vi "Write Slow FPGA Telem to FIFO.vi"   [LabVIEW 2015]
uses:
  FPGA Telem for Slow Logging.ctl
  <vilib>/FPGAPlugInAG/Dynamic/niLvFpga_Close_Dynamic.vi
  <vilib>/rvi/errors/niLvFpgaAdjustHostInterfaceError.vi
  <vilib>/Utility/error.llb/Error Cluster From Error Code.vi
  Global Data.vi
  <vilib>/rvi/interface/common/dynamic/niFpgaDynamicAddResources.vi
  <vilib>/FPGAPlugInAG/sbRIO-9627/niLvFpga_Open_sbRIO-9627.vi
  <vilib>/rvi/interface/nirviCloseFPGA/nirviCloseFPGA.xnode
  <vilib>/rvi/interface/nirviReadWriteControl/nirviReadWriteControl.xnode
  <vilib>/rvi/interface/nirviOpenFPGA/nirviOpenFPGA.xnode
  FPGA Bitfiles/Latest.lvbitx
  <vilib>/NI_Real-Time Target Support.lvlib
  NiFpgaLv.dll
  <vilib>/rvi/interface/Simulation/niFpgaSimulationCallBeginRW.vi
types:
  T1 = cluster{"read mode":enum16{"polling", "blocking"}, "write mode":enum16{"polling", "blocking"}}
  T2 = typedef "FPGA Telem for Slow Logging.ctl" = cluster{"TSBRIO":fxp<+/-,16,9>, "VsbRIOSpply":fxp<+/-,25,6>, "bFPGALED":bool, "CPU Load":cluster{"Total (%)":dbl, "Time Critical (%)":dbl, "Timed Structures (%)":dbl, "High (%)":dbl, "Above Normal (%)":dbl, "Normal (%)":dbl, "Background (%)":dbl, "Idle (%)":dbl, "ISR (%)":dbl}, "Time Stamp":timestamp, "NLatiPhone":dbl, "NLongiPhone":dbl, "nGPSiPhone":dbl, "IHighCurrent":fxp<+/-,24,15>, "ILowCurrent":fxp<+/-,24,15>, "V5VSupply":fxp<+/-,24,5>, "tCurrentLap":u32, "tLastLap":u32, "NLap":u8, "bCoolantPumpEnable":bool, "bRTDSEnable":bool, "bTSMSInStatus":bool, "bPosAIREnable":bool, "bBMSOK":bool, "bIMDOK":bool, "bBSPDOK":bool, "bSBRIOOK2":bool, "bSBRIOOK1":bool, "bTSMSOutStatus":bool, "bMotorControllerEnable":bool, "Tire Diameter(m)":fxp<+,16,1>}
  T3 = typedef "NI_Real-Time Target Support.lvlib/RT CPU Load.ctl" = cluster{"Total (%)":dbl, "Time Critical (%)":dbl, "Timed Structures (%)":dbl, "High (%)":dbl, "Above Normal (%)":dbl, "Normal (%)":dbl, "Background (%)":dbl, "Idle (%)":dbl, "ISR (%)":dbl}
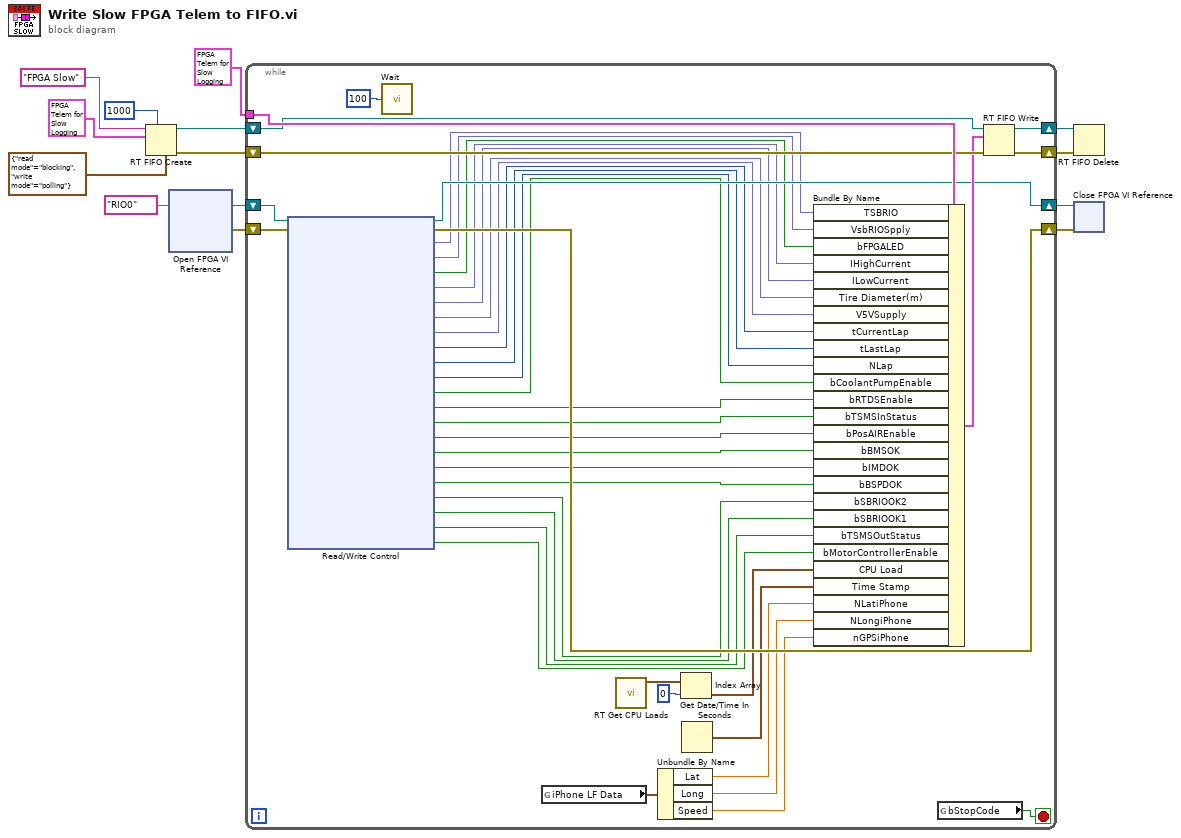
[diagram p0: block diagram]
diagram:
  n1 = RT FIFO Create(0:"FPGA Slow" ("name (unnamed)"), 1:T2 {"TSBRIO"=0.0, "VsbRIOSpply"=0.0, "bFPGALED"=FALSE, "CPU Load"={"Total (%)"=0.0, "Time Critical (%)"=0.0, "Timed Structures (%)"=0.0, "High (%)"=0.0, "Above Normal (%)"=0.0, "Normal (%)"=0.0, "Background (%)"=0.0, "Idle (%)"=0.0, "ISR (%)"=0.0}, "Time Stamp"=timestamp(0 s since 1904-01-01), "NLatiPhone"=0.0, "NLongiPhone"=0.0, "nGPSiPhone"=0.0, "IHighCurrent"=0.0, "ILowCurrent"=0.0, "V5VSupply"=-16.0, "tCurrentLap"=4, "tLastLap"=0, "NLap"=0, "bCoolantPumpEnable"=FALSE, "bRTDSEnable"=FALSE, "bTSMSInStatus"=FALSE, "bPosAIREnable"=FALSE, "bBMSOK"=TRUE, "bIMDOK"=TRUE, "bBSPDOK"=FALSE, "bSBRIOOK2"=FALSE, "bSBRIOOK1"=FALSE, "bTSMSOutStatus"=FALSE, "bMotorControllerEnable"=FALSE, "Tire Diameter(m)"=0.0} ("FPGA Logging Telem"), 4:u32 1000 ("size (10)"), 7:T1 {"read mode"=enum."blocking", "write mode"=enum."polling"} ("r/w modes (polling,polling)")) -> (8:w7:refnum<k33>, 11:w6:errorcluster)  [unwired: 4 in, 1 out]
  n2 = xnode "Open FPGA VI Reference"("resource name"=tag "RIO0") -> ("FPGA VI Reference Out"=w13:refnum<k20>, "error out"=w12:errorcluster)  [unwired: 1 in]
  n3 = while {
    tunnel: T2 {"TSBRIO"=0.0, "VsbRIOSpply"=0.0, "bFPGALED"=FALSE, "CPU Load"={"Total (%)"=0.0, "Time Critical (%)"=0.0, "Timed Structures (%)"=0.0, "High (%)"=0.0, "Above Normal (%)"=0.0, "Normal (%)"=0.0, "Background (%)"=0.0, "Idle (%)"=0.0, "ISR (%)"=0.0}, "Time Stamp"=timestamp(0 s since 1904-01-01), "NLatiPhone"=0.0, "NLongiPhone"=0.0, "nGPSiPhone"=0.0, "IHighCurrent"=0.0, "ILowCurrent"=0.0, "V5VSupply"=-16.0, "tCurrentLap"=4, "tLastLap"=0, "NLap"=0, "bCoolantPumpEnable"=FALSE, "bRTDSEnable"=FALSE, "bTSMSInStatus"=FALSE, "bPosAIREnable"=FALSE, "bBMSOK"=TRUE, "bIMDOK"=TRUE, "bBSPDOK"=FALSE, "bSBRIOOK2"=FALSE, "bSBRIOOK1"=FALSE, "bTSMSOutStatus"=FALSE, "bMotorControllerEnable"=FALSE, "Tire Diameter(m)"=0.0} ("FPGA Logging Telem") -> [w55]
    shift-right: [w47] -> w4
    shift-left: w7 -> [w50]
    shift-right: [w46] -> w5
    shift-left: w6 -> [w49]
    shift-right: [w44] -> w3
    shift-left: w13 -> [w54]
    shift-right: [w43] -> w2
    shift-left: w12 -> [w53]
    stop <- w28 stop-if-true
    n4 = xnode "Read/Write Control"("FPGA VI Reference In"=w54, "error in"=w53) -> ("FPGA VI Reference Out"=w44:refnum<k20>, "error out"=w43:errorcluster, "TSBRIO"=w41:fxp<+,19,8>, "VsbRIOSupply"=w40:fxp<+/-,25,6>, "bFPGALED"=w39:bool, "IHighCurrent"=w38:fxp<+/-,19,15>, "ILowCurrent"=w37:fxp<+/-,19,15>, "Tire Diameter(m)"=w26:fxp<+,16,1>, "V5VSupply"=w36:fxp<+/-,24,5>, "tCurrentLap"=w35:u32, "tLastLap"=w34:u32, "NLap"=w27:u8, "bCoolantPumpEnable"=w25:bool, "bRTDSEnable"=w24:bool, "bTSMSInStatus"=w23:bool, "bPosAIREnable"=w22:bool, "bBMSOK"=w21:bool, "bIMDOK"=w20:bool, "bBSPDOK"=w19:bool, "bSBRIOOK2"=w18:bool, "bSBRIOOK1"=w17:bool, "bTSMSOutStatus"=w16:bool, "bMotorControllerEnable"=w15:bool)
    n5 = call "Wait"("Count(mSec)"=u32 100) -> ()  [unwired: 1 out]
    n6 = global read "Global Data.vi" "iPhone LF Data"() -> (w42:cluster{"Lat":dbl, "Long":dbl, "Speed":dbl})
    n7 = call <vilib>:"RT Get CPU Loads.vi"() -> ("CPU loads"=w52:T3[])  [unwired: 10 in, 1 out]
    n8 = Unbundle By Name(w42) -> ("Lat"=w31:dbl, "Long"=w30:dbl, "Speed"=w29:dbl)
    n9 = Index Array(array=w52, index=0) -> (element=w33:T3)
    n10 = Get Date/Time In Seconds() -> (seconds since 1Jan1904=w32:timestamp)
    n11 = Bundle By Name(cluster=w55, "TSBRIO"=w41, "VsbRIOSpply"=w40, "bFPGALED"=w39, "IHighCurrent"=w38, "ILowCurrent"=w37, "Tire Diameter(m)"=w26, "V5VSupply"=w36, "tCurrentLap"=w35, "tLastLap"=w34, "NLap"=w27, "bCoolantPumpEnable"=w25, "bRTDSEnable"=w24, "bTSMSInStatus"=w23, "bPosAIREnable"=w22, "bBMSOK"=w21, "bIMDOK"=w20, "bBSPDOK"=w19, "bSBRIOOK2"=w18, "bSBRIOOK1"=w17, "bTSMSOutStatus"=w16, "bMotorControllerEnable"=w15, "CPU Load"=w33, "Time Stamp"=w32, "NLatiPhone"=w31, "NLongiPhone"=w30, "nGPSiPhone"=w29) -> (w48:T2)
    n12 = global read "Global Data.vi" "bStopCode"() -> (w28:bool)
    n13 = RT FIFO Write(0:w50, 1:w48, 3:w49) -> (8:w47:refnum<k33>, 11:w46:errorcluster)  [unwired: 2 in, 2 out]
  }
  n14 = RT FIFO Delete(0:w4, 3:w5) -> ()  [unwired: 1 in, 1 out]
  n15 = xnode "Close FPGA VI Reference"("FPGA VI Reference In"=w3, "error in"=w2) -> ()  [unwired: 1 out]
